vi "Step ADD DCW W Parameters.vi"(0 "VISA resource name":refnum<visa-resource-name>, 1 "Scanner Settings":T2={"Scan1"=1, "Scan2"=1, "Scan3"=1, "Scan4"=1, "Scan5"=1, "Scan6"=1, "Scan7"=1, "Scan8"=1, "Scan9"=1, "Scan10"=1, "Scan11"=1, "Scan12"=1, "Scan13"=1, "Scan14"=1, "Scan15"=1, "Scan16"=1} {"Scan16" scale=0.0..2.0; "Scan15" scale=0.0..2.0; "Scan14" scale=0.0..2.0; "Scan13" scale=0.0..2.0; "Scan12" scale=0.0..2.0; "Scan11" scale=0.0..2.0; "Scan10" scale=0.0..2.0; "Scan9" scale=0.0..2.0; "Scan8" scale=0.0..2.0; "Scan7" scale=0.0..2.0; "Scan6" scale=0.0..2.0; "Scan5" scale=0.0..2.0; "Scan4" scale=0.0..2.0; "Scan3" min=0 max=2 scale=0.0..2.0; "Scan2" min=0 max=2 scale=0.0..2.0; "Scan1" min=0 max=2 scale=0.0..2.0}, 2 "Internal scanner?":bool, 5 "DCW Test Parameters (in)":T1={"Voltage (0~6.0 KV)"=1.0, "High Limit(0.0~7500 uA)"=10.0, "Low Limit(0~7500 uA)"=0.0, "Ramp Up Time (0.1~999.9 seconds)"=0.1, "Dwell Time (0, 0.4~999.9 seconds)"=1.0, "Ramp Down Time (0, 1.0~999.9 seconds)"=0.0, "Charge LO (0.0~350uA)"=0.0, "Arc Sense (1~9)"=5, "Arc Detect (F: Off)"=FALSE, "Auto Charge LO (F: Off)"=FALSE, "Ramp-Hi (0.0~7500 uA)"=0.0} {"Ramp-Hi (0.0~7500 uA)" format="%.2f"; "Ramp Down Time (0, 1.0~999.9 seconds)" format="%.1f"; "Charge LO (0.0~350uA)" format="%.2f"; "Dwell Time (0, 0.4~999.9 seconds)" format="%.1f"; "Ramp Up Time (0.1~999.9 seconds)" format="%.1f"; "Low Limit(0~7500 uA)" format="%.1f"; "High Limit(0.0~7500 uA)" format="%.2f"; "Voltage (0~6.0 KV)" format="%.1f"}, 7 "Step Selection (1-200)":i32=1, 9 "Add Step":bool, 11 "error in (no error)":errorcluster) -> (4 "VISA resource name out":refnum<visa-resource-name>, 15 "error out":errorcluster)   [LabVIEW 2016, in "eec EST 300.lvlib"]
doc: "Inserts a DCW test with the User defined parameters into the assigned Step Selecton.\n\nIf Add step is set to Edit, it will replace the existing step. If it is set to Add it will insert the new step and increment all steps after the selected step by 1.\n\nSee specifications for Limits."
uses:
  <instrlib>/eec EST 300/eec EST 300.lvlib
  <instrlib>/eec EST 300/Public/Configure/Steps/Low Level/Scanner Settings.ctl
  <instrlib>/eec EST 300/Public/Configure/Steps/Low Level/DCW Test Parameters.ctl
panel:
  # "Add"
  # "Edit"
  # "On\nOff"
  # "On\nOff"
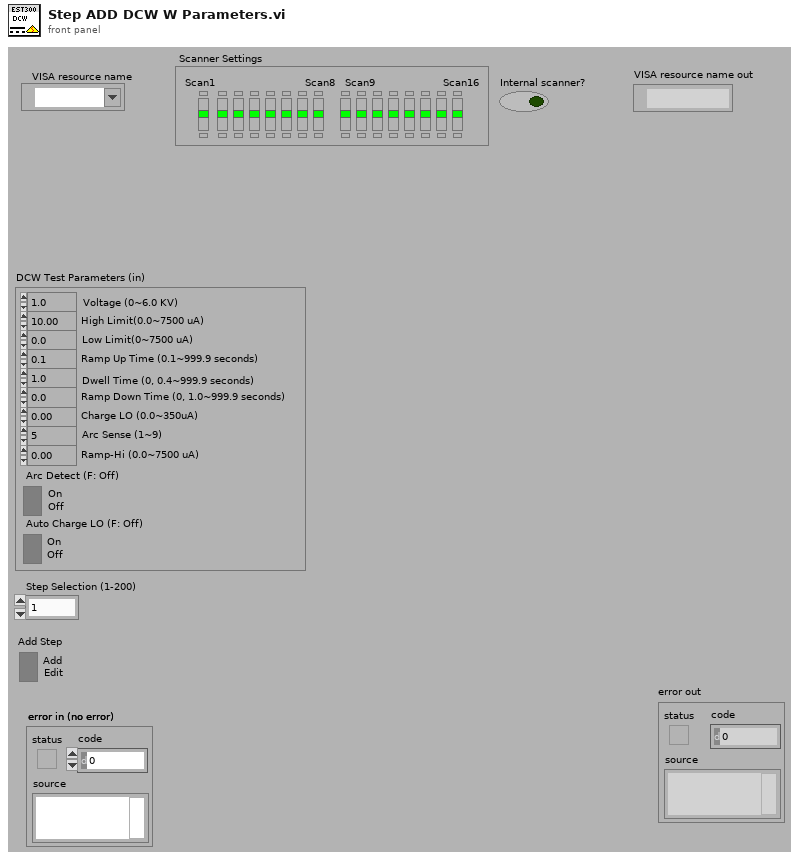
[diagram p1: front panel]
types:
  T1 = typedef "eec EST 300.lvlib/DCW Test Parameters.ctl" = cluster{"Voltage (0~6.0 KV)":dbl, "High Limit(0.0~7500 uA)":dbl, "Low Limit(0~7500 uA)":dbl, "Ramp Up Time (0.1~999.9 seconds)":dbl, "Dwell Time (0, 0.4~999.9 seconds)":dbl, "Ramp Down Time (0, 1.0~999.9 seconds)":dbl, "Charge LO (0.0~350uA)":dbl, "Arc Sense (1~9)":i32, "Arc Detect (F: Off)":bool, "Auto Charge LO (F: Off)":bool, "Ramp-Hi (0.0~7500 uA)":dbl}
  T2 = typedef "eec EST 300.lvlib/Scanner Settings.ctl" = cluster{"Scan1":i32, "Scan2":i32, "Scan3":i32, "Scan4":i32, "Scan5":i32, "Scan6":i32, "Scan7":i32, "Scan8":i32, "Scan9":i32, "Scan10":i32, "Scan11":i32, "Scan12":i32, "Scan13":i32, "Scan14":i32, "Scan15":i32, "Scan16":i32}
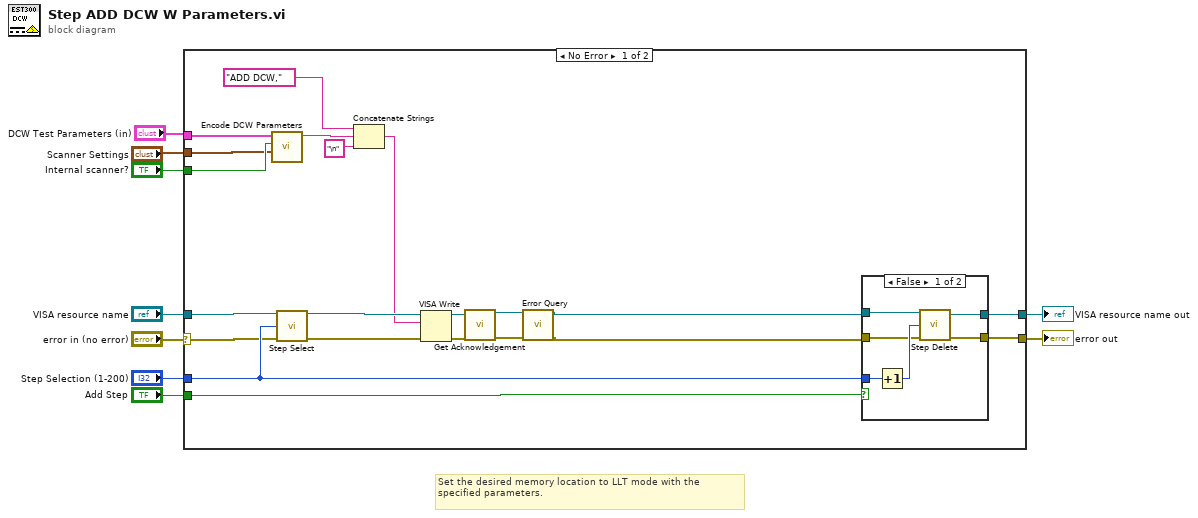
[diagram p0: block diagram]
diagram:
  # "Set the desired memory location to LLT mode with the specified parameters."
  n1 = case shown="No Error" "error in (no error)" {
    selector: "error in (no error)" -> [w19 w40]
    tunnel: [w28 w40] -> w8
    tunnel: [w27 w39] -> w6
    tunnel: "VISA resource name" -> [w20 w39]
    tunnel: "Step Selection (1-200)" -> [w21 _]
    tunnel: "Add Step" -> [w26 _]
    tunnel: "Scanner Settings" -> [w13 _]
    tunnel: "Internal scanner?" -> [w15 _]
    tunnel: "DCW Test Parameters (in)" -> [w12 _]
    frame No Error {
      n2 = call <instrlib>:"Encode DCW Parameters.vi"("Scanner Settings In"=w13, "Internal Scanner Exists?"=w15, "DCW Test Parameters (in)"=w12) -> ("Add Parameters"=w14:string)  [unwired: 6 in, 2 out]
      n3 = call <instrlib>:"Step Select.vi"("VISA resource name"=w20, "Step Number (1)"=w21, "error in (no error)"=w19) -> ("VISA resource name out"=w29:refnum<visa-resource-name>, "error out"=w30:errorcluster)  [unwired: 11 in]
      n4 = Concatenate Strings("ADD DCW," ("string"), w14, "\n" ("string")) -> (w24:string)
      n5 = VISA Write(VISA resource name=w29, write buffer=w24, error in (no error)=w30) -> (VISA resource name out=w17:refnum<visa-resource-name>, error out=w16:errorcluster)  [unwired: 1 out]
      n6 = call <instrlib>:"Get Acknowledgement.vi"("VISA resource name"=w17, "error in (no error)"=w16) -> ("VISA resource name out"=w23:refnum<visa-resource-name>, "error out"=w22:errorcluster)  [unwired: 12 in]
      n7 = call <instrlib>:"Error Query.vi"("VISA resource name"=w23, "error in (no error)"=w22) -> ("VISA resource name out"=w11:refnum<visa-resource-name>, "error out"=w10:errorcluster)  [unwired: 10 in, 2 out]
      n8 = case shown="False" w26 {
        tunnel: w21 -> [w36 _]
        tunnel: w10 -> [w34 w37]
        tunnel: w11 -> [w33 w38]
        tunnel: [w32 w37] -> w28
        tunnel: [w31 w38] -> w27
        frame False {
          n9 = Increment(x=w36) -> (x+1=w35:i32)
          n10 = call <instrlib>:"Step Delete.vi"("VISA resource name"=w33, "Step Number (0 = Active Step)"=w35, "error in (no error)"=w34) -> ("VISA resource name out"=w31:refnum<visa-resource-name>, "error out"=w32:errorcluster)  [unwired: 11 in]
        }
        frame True {
        }
      }
    }
    frame Error {
    }
  }
  "error out" <- w8
  "VISA resource name out" <- w6
